vi "getConfigElement.vi"(2 "element":string="localport", 3 "all rows":string[][](array[string])) -> (0 "error in":errorcluster, 1 "value":string)   [LabVIEW 2009]
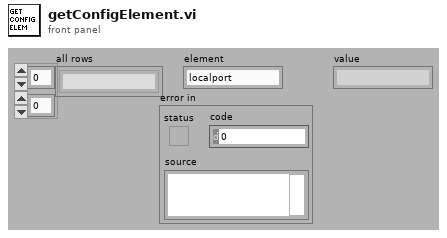
[diagram p1: front panel]
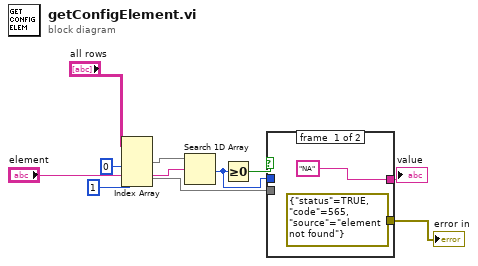
[diagram p0: block diagram]
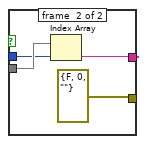
[diagram p2: hidden frame]
diagram:
  n1 = Index Array(array="all rows", index (col) #1=0 ("disabled index (col)"), index (col) #2=1 ("index (col)")) -> (element #1=w4:string[], element #2=w8:string[])  [unwired: 2 in]
  n2 = Search 1D Array(1D array=w4, element="element") -> (index of element=w9:i32)  [unwired: 1 in]
  n3 = Greater Or Equal To 0?(x=w9) -> (x >= 0?=w6:bool)
  n4 = case shown="True" w6 {
    tunnel: w8 -> [_ w16]
    tunnel: w9 -> [_ w15]
    tunnel: ["NA" ("String") w14] -> w10
    tunnel: [errorcluster {"status"=TRUE, "code"=565, "source"="element not found"} ("error in") errorcluster {"status"=FALSE, "code"=0, "source"=""} ("error in")] -> w1
    frame #0 {
    }
    frame #1 {
      n5 = Index Array(array=w16, index=w15) -> (element=w14:string)
    }
  }
  "value" <- w10
  "error in" <- w1
